vi "5.7-UDP Make Checksum.vi"(0 "Data String In":string) -> (1 "CS String Out":string, 2 "Sum":u8)   [LabVIEW 2010]
doc: "Creates a simple u8 checksum and prepends it to the string. Used to prevent use of mistransmitted data over UDP"
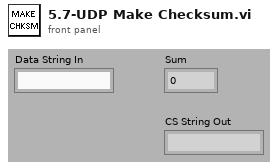
[diagram p1: front panel]
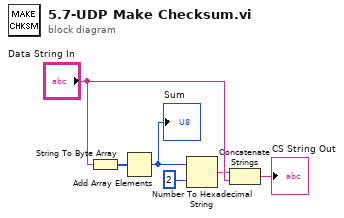
[diagram p0: block diagram]
diagram:
  n1 = String To Byte Array(string="Data String In") -> (unsigned byte array=w1:u8[])
  n2 = Add Array Elements(numeric array=w1) -> (sum=w2:u8)
  "Sum" <- w2
  n3 = Number To Hexadecimal String(1:i16 2 ("width (-)"), 2:w2) -> (0:w3:string)
  n4 = Concatenate Strings(w3, "Data String In") -> (→"CS String Out":string)
